vi "Write Settings XML.vi"(8 "error in (no error)":errorcluster, 11 "path":path) -> (0 "error out":errorcluster, 3 "XML File Path(duplicate)":path)   [LabVIEW 2020]
uses:
  _controls/OpticalPrime Ctrls For Saving.ctl
  _controls/Exp Params.ctl
  _controls/Ventus Control.ctl
  _controls/xiCam.ctl
  <vilib>/userDefined/High Color/IMAQdx.ctl
  _controls/Spot Params.ctl
  _controls/PCIe SLM params.ctl
  _globals/OpticalPrime Controls.vi
  <vilib>/Utility/xml.llb/Write to XML File(string).vi
panel:
  out "XML String":string
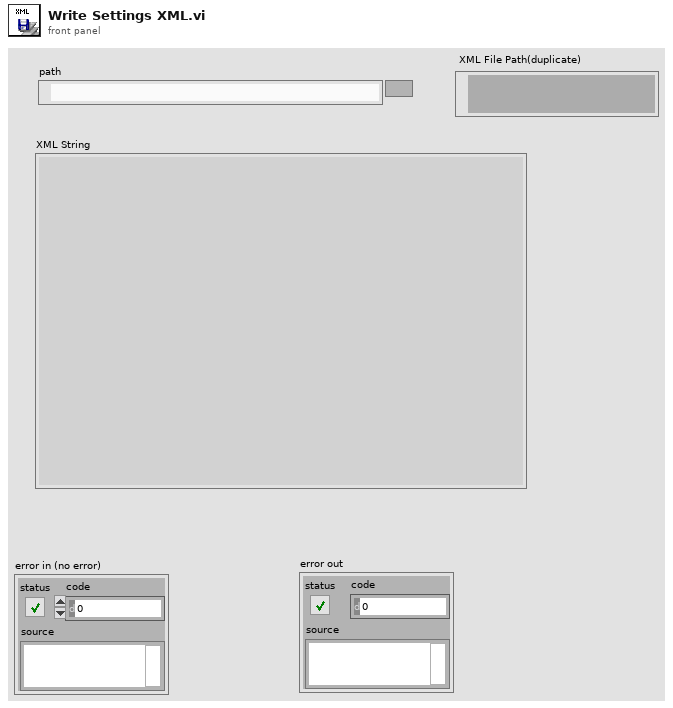
[diagram p1: front panel]
types:
  T1 = typedef "OpticalPrime Ctrls For Saving.ctl" = cluster{"Time Stamp":cluster{"date string":string, "time string":string}, "Exp Params":T2, "Ventus Controls":T3, "Camera Controls":T4, "Spot Params":T6, "SLM Parameters":T7}
  T2 = typedef "Exp Params.ctl" = cluster{"Experiment Type":string, "Experiment Name":string, "ExpPath":path, "Save As":string, "TSFrames":i32, "TSfps":dbl, "Streaming":bool, "tdms ref":refnum<k34>, "frame #":i64, "Full Path":path, "PeakOnQueue":bool}
  T3 = typedef "Ventus Control.ctl" = cluster{"Ventus Power":dbl, "Open Serial":bool, "VISA Refnum":refnum<visa-resource-name>}
  T4 = typedef "xiCam.ctl" = cluster{"Exposure Time (ms)":u32, "cam0 Session":T5, "Camera ROI":cluster{"Width":u32, "Height":u32, "Offset X":u32, "Offset Y":u32}, "Command":string}
  T5 = typedef "IMAQdx.ctl" = refnum<k21>
  T6 = typedef "Spot Params.ctl" = cluster{"Intensity":dbl, "Vortex":dbl, "Phase":dbl, "X":dbl, "Y":dbl, "Z":dbl}[]
  T7 = typedef "PCIe SLM params.ctl" = cluster{"Width":dbl, "Height":dbl, "Board ID":i32, "Centre Y":dbl, "Centre X":dbl}
  T8 = typedef "OpticalPrime Ctrl Refs.ctl" = cluster{"Exp Params":refnum<vi>, "Ventus Controls":refnum<vi>, "SLM Parameters":refnum<vi>, "Spot Params":refnum<vi>, "Camera Controls":refnum<vi>}
  T9 = cluster{"date string":string, "time string":string}
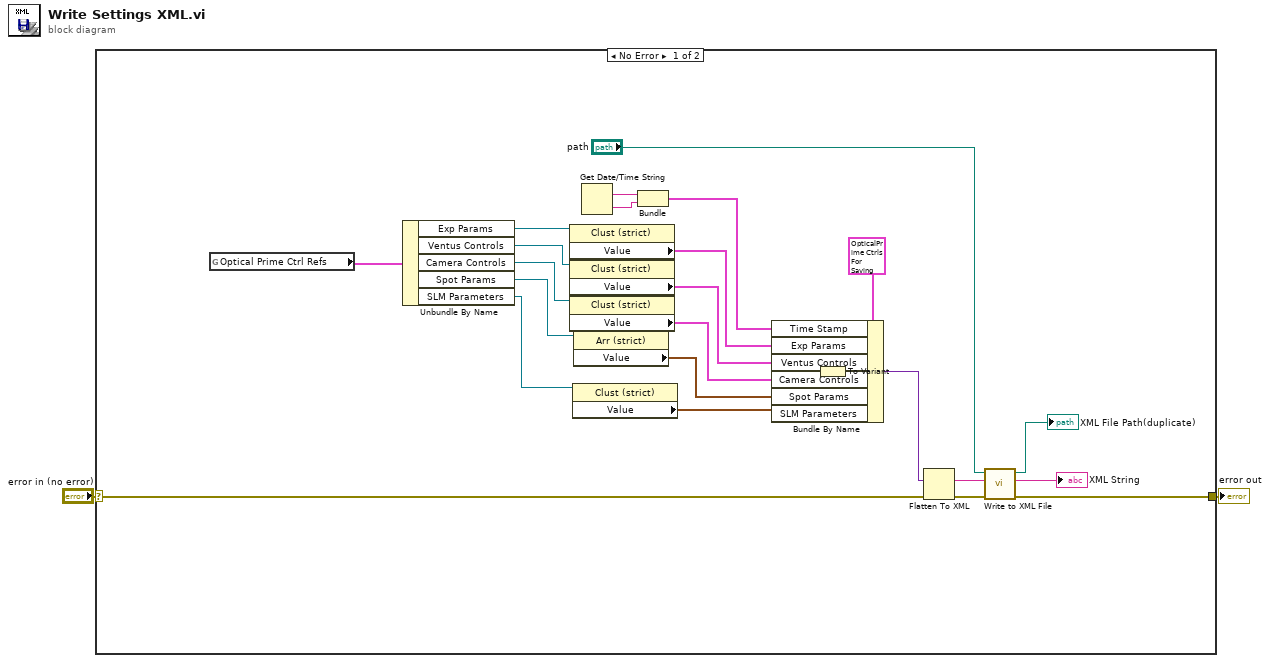
[diagram p0: block diagram]
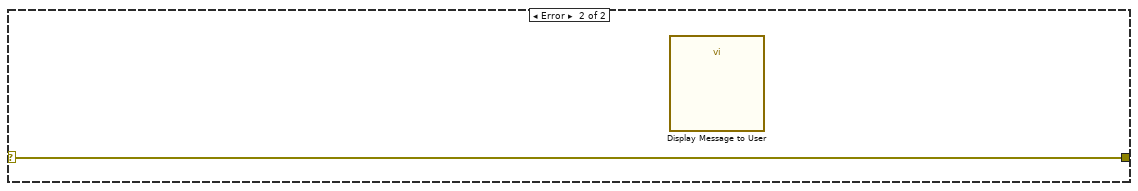
[diagram p2: hidden frame]
diagram:
  n1 = case shown="No Error" "error in (no error)" {
    selector: "error in (no error)" -> [w25 w26]
    tunnel: [w22 w26] -> w1
    frame No Error {
      n2 = global read "OpticalPrime Controls.vi" "Optical Prime Ctrl Refs"() -> (w11:T8)
      n3 = Unbundle By Name(w11) -> ("Exp Params"=w19:refnum<vi>, "Ventus Controls"=w20:refnum<vi>, "Camera Controls"=w21:refnum<vi>, "Spot Params"=w13:refnum<vi>, "SLM Parameters"=w7:refnum<vi>)
      n4 = property on="Property Node" class="Clust (strict)"(reference=w19) -> ("Value"=w16:T2)  [unwired: 1 in, 2 out]
      n5 = property on="Property Node" class="Clust (strict)"(reference=w20) -> ("Value"=w18:T3)  [unwired: 1 in, 2 out]
      n6 = property on="Property Node" class="Clust (strict)"(reference=w21) -> ("Value"=w17:T4)  [unwired: 1 in, 2 out]
      n7 = property on="Property Node" class="Clust (strict)"(reference=w7) -> ("Value"=w6:T7)  [unwired: 1 in, 2 out]
      n8 = property on="Property Node" class="Arr (strict)"(reference=w13) -> ("Value"=w12:T6)  [unwired: 1 in, 2 out]
      n9 = Get Date/Time String() -> (date string=w10:string, time string=w9:string)  [unwired: 3 in]
      n10 = Bundle("date string"=w10, "time string"=w9) -> (w8:T9)  [unwired: 1 in]
      n11 = Bundle By Name(cluster=T1 {"Time Stamp"={"date string"="", "time string"=""}, "Exp Params"={"Experiment Type"="Time Series", "Experiment Name"="Experiment_1", "ExpPath"=path "D:/Data", "Save As"="TIFF", "TSFrames"=1000, "TSfps"=1.0, "Streaming"=TRUE, "tdms ref"=refnum, "frame #"=0, "Full Path"=path "", "PeakOnQueue"=FALSE}, "Ventus Controls"={"Ventus Power"=0.0, "Open Serial"=FALSE, "VISA Refnum"=""}, "Camera Controls"={"Exposure Time (ms)"=27, "cam0 Session"="", "Camera ROI"={"Width"=0, "Height"=0, "Offset X"=0, "Offset Y"=0}, "Command"=""}, "Spot Params"=[], "SLM Parameters"={"Width"=0.0, "Height"=0.0, "Board ID"=0, "Centre Y"=0.0, "Centre X"=0.0}} ("OpticalPrime Ctrls For Saving"), "Time Stamp"=w8, "Exp Params"=w16, "Ventus Controls"=w18, "Camera Controls"=w17, "Spot Params"=w12, "SLM Parameters"=w6) -> (w15:T1)
      n12 = To Variant(anything=w15) -> (Variant=w14:variant)
      n13 = Flatten To XML(6:w14) -> (2:w23:string)
      n14 = call-poly <vilib>:"Write to XML File.vi"("error in (no error)"=w25, "XML Input"=w23, "XML File Path"="path") -> ("error out"=w22:errorcluster, "XML String"=→"XML String":string, "XML File Path(duplicate)"=→"XML File Path(duplicate)":path)  [unwired: 6 in]
    }
    frame Error {
      n15 = call "Display Message to User"() -> ()  [unwired: 10 in, 2 out]
    }
  }
  "error out" <- w1
